vi "Write Motion Magic Constants.vi"(8 "error in (no error)":errorcluster, 10 "Motion Magic Constants":T1, 11 "Drive in":refnum<class "Drive.lvclass">) -> (0 "error out":errorcluster, 3 "Drive out":refnum<class "Drive.lvclass">)   [LabVIEW 2019, in "DriveOld.lvlib" / "Drive.lvclass"]
uses:
  Drive.lvclass
  Controls/Motion Magic Constants.ctl
  Drive.lvclass/Drive.ctl
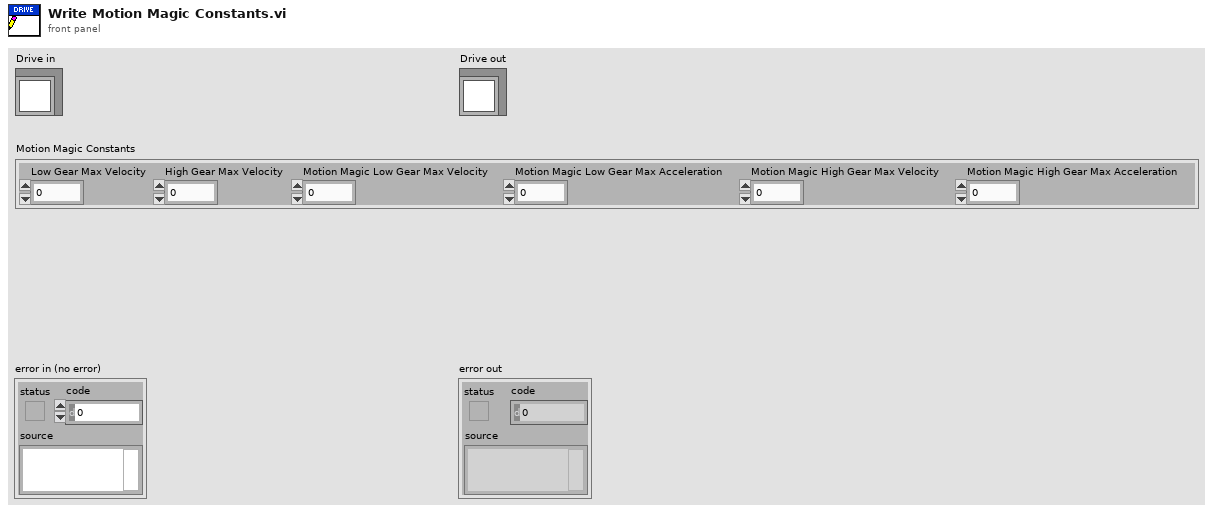
[diagram p1: front panel]
types:
  T1 = typedef "DriveOld.lvlib/Drive.lvclass/Motion Magic Constants.ctl" = cluster{"Low Gear Max Velocity":u32, "High Gear Max Velocity":u32, "Motion Magic Low Gear Max Velocity":u32, "Motion Magic Low Gear Max Acceleration":u32, "Motion Magic High Gear Max Velocity":u32, "Motion Magic High Gear Max Acceleration":u32}
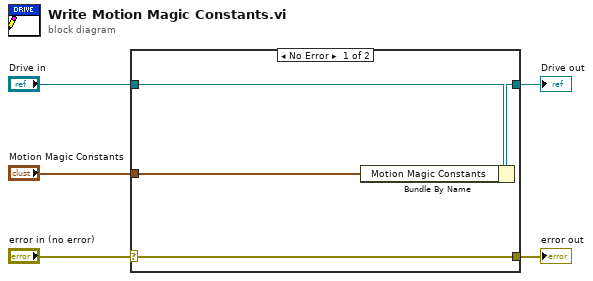
[diagram p0: block diagram]
diagram:
  n1 = case shown="No Error" "error in (no error)" {
    selector: "error in (no error)" -> [w9 w10]
    tunnel: [w9 w10] -> w4
    tunnel: [w7 w11] -> w2
    tunnel: "Drive in" -> [w8 w11]
    tunnel: "Motion Magic Constants" -> [w6 _]
    frame No Error {
      n2 = Bundle By Name(cluster=w8, "Motion Magic Constants"=w6) -> (w7:refnum<class "Drive.lvclass">)
    }
    frame Error {
    }
  }
  "error out" <- w4
  "Drive out" <- w2
